vi "OJ-Pick Up Test.vi"   [LabVIEW 2020]
uses:
  Classes/Routine/Pick and Place/Pick and Place.lvclass
  Classes/Routine/Pick and Place/Pick and Place Type.ctl
  Classes/Workspace/Pick Up Tool Area/Pick Up Tool Fixture.lvclass
  Classes/Routine/Pick and Place/Pick and Place.lvclass/Pick and Place.ctl
  Classes/Routine/Pick and Place/Write Pick and Place Type.vi
  Classes/Controller/Controller.lvclass
types:
  T1 = typedef "Pick and Place.lvclass/Pick and Place Type.ctl" = enum16{"Primary Pick Up", "Secondary Pick Up", "Put Down All", "Pick Up All", "Put Down Secondary"}
  T2 = typedef "Controller.lvclass/Controllers.ctl" = cluster{"I-O.lvclass":refnum<class "I-O.lvclass">, "Dispenser.lvclass":refnum<class "Dispenser.lvclass">, "Gantry":refnum<k24>}
  T3 = typedef "Fixture.lvclass/Workspace.ctl" = cluster{"XYZTheta":dbl[], "Workspace Valve":i32, "Workspace Sensor":i32}
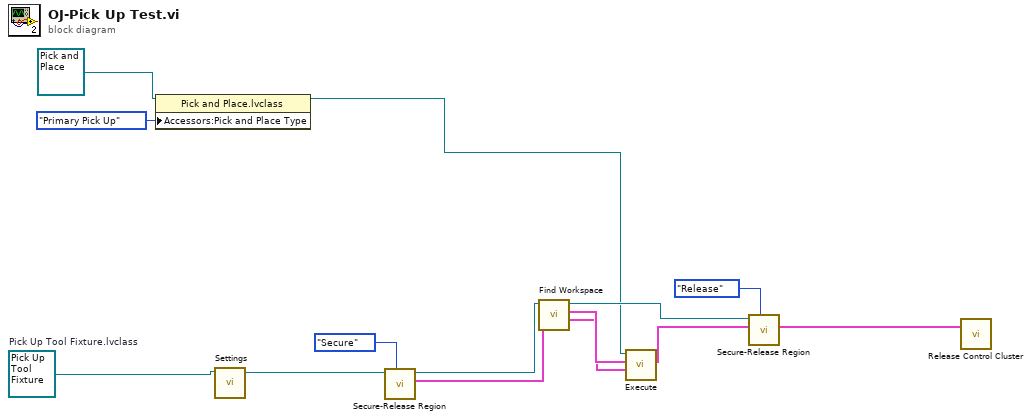
[diagram p0: block diagram]
diagram:
  w12 = refnum<class "Pick Up Tool Fixture.lvclass"> refnum  # Pick Up Tool Fixture.lvclass
  n1 = property class="Pick and Place.lvclass"(reference=refnum<class "Pick and Place.lvclass"> refnum ("Pick and Place.lvclass"), "Accessors:Pick and Place Type"=Pick_and_Place_Type."Primary Pick Up" ("Pick and Place Type")) -> (reference out=w3:refnum<class "Pick and Place.lvclass">)  [unwired: 1 in, 1 out]
  n2 = call-dynamic "Settings.vi"("Workspace in"=w12) -> ("Workspace out"=w11:refnum<class "Pick Up Tool Fixture.lvclass">)  [unwired: 9 in, 1 out]
  n3 = call-dynamic "Secure-Release Region.vi"("Action"=enum16{"Secure", "Release"}."Secure", "Fixture in"=w11) -> ("Control Out"=w8:T2, "Fixture out"=w9:refnum<class "Pick Up Tool Fixture.lvclass">)  [unwired: 7 in, 1 out]
  n4 = call-dynamic "Find Workspace.vi"("Control In"=w8, "Workspace In"=w9) -> (1:"Workspace Out"=w5:T3, "Control Out"=w6:T2, 3:"Workspace Out"=w7:refnum<class "Pick Up Tool Fixture.lvclass">)  [unwired: 6 in, 1 out]
  n5 = call-dynamic "Execute.vi"("Workspace"=w5, "Cluster"=w6, "Pick and Place in"=w3) -> ("Control Out"=w4:T2)  [unwired: 6 in, 2 out]
  n6 = call-dynamic "Secure-Release Region.vi"("Action"=enum16{"Secure", "Release"}."Release", "Control In"=w4, "Fixture in"=w7) -> ("Control Out"=w2:T2)  [unwired: 6 in, 2 out]
  n7 = call "Release Control Cluster.vi"("output cluster"=w2) -> ()  [unwired: 11 in]
